vi "spectrum-voice.vi"() -> ()   [LabVIEW 2016]
doc: "This VI configures your sound card for both input and output. On a Macintosh, it could be the same device, while on Windows, it has to be different. Because of the delay of data buffering, it creates an effect of echoing."
uses:
  <vilib>/sound2/lvsound2.llb/Sound Data Format.ctl
  <vilib>/Analysis/3filter.llb/IIR Cascade Filter with I.C. (DBL).vi
  <vilib>/sound2/lvsound2.llb/Sound Input Read (DBL).vi
  <vilib>/express/express analysis/Spectral/Block/exnSpectralBlock spectral measurements power poly.vi
  <vilib>/express/express analysis/Spectral/Block/exnSpectralBlock spectral measurements power DDT.vi
  <vilib>/sound2/lvsound2.llb/Sound Output Write (DBL Single).vi
  <vilib>/express/express analysis/Spectral/XNode/ExpressSpectralMeasurementsBlockNode.xnode
  <vilib>/Analysis/NI_AALBase.lvlib
panel:
  in  "device ID":u32
  in  "Microphone\nAmplification":dbl(knob)=24.0 scale=0.0..100.0
  out "Time-Domain (Oscilloscope) Display":waveform(dbl)(graph)
  out "Frequency Display":dynamicdata(graph)
  in  "Filter":bool
  in  "filter type":T1(ring)
  in  "stop":bool
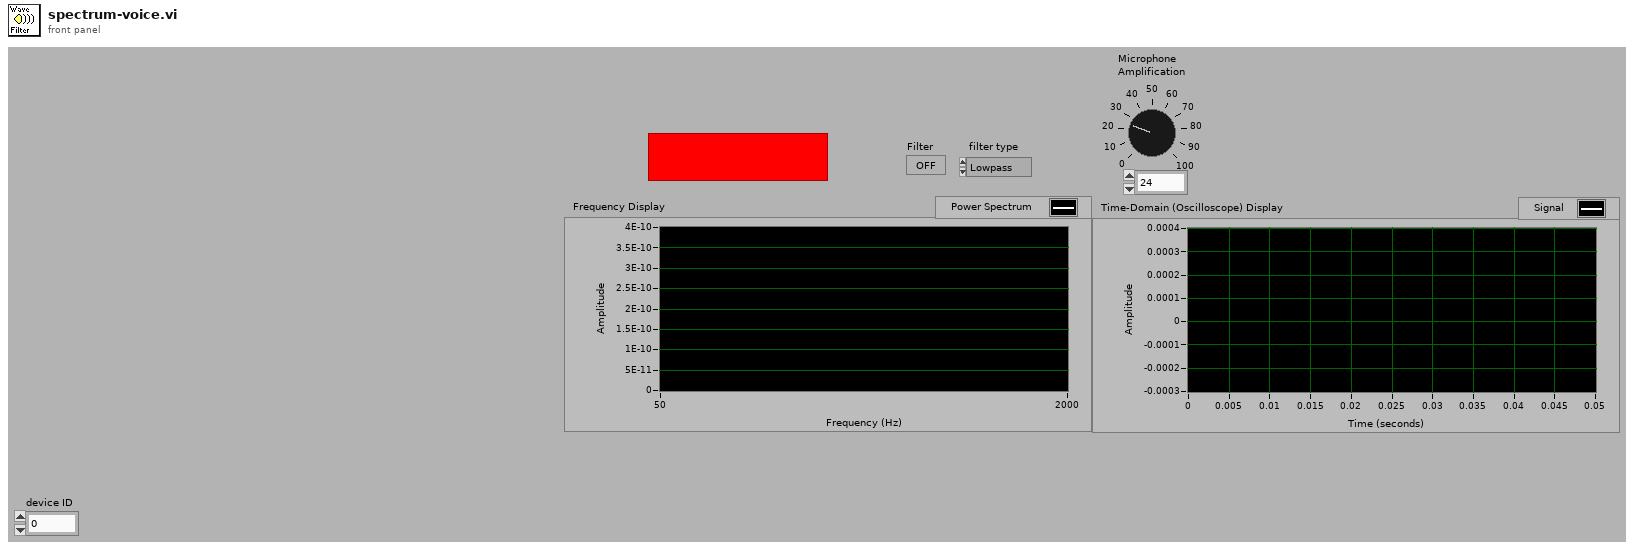
[diagram p1: front panel]
types:
  T1 = enum32{"Lowpass", "Highpass", "Bandpass", "Bandstop"}
  T2 = typedef "Sound Data Format.ctl" = cluster{"sample rate (S/s)":dbl, "number of channels":i32, "bits per sample":i32}
  T3 = typedef "Sound Output Task ID.ctl" = u32
  T4 = typedef "Sound Input Task ID.ctl" = u32
  T5 = cluster{"averaging mode":u16, "weighting mode":u16, "number of averages":u32}
  T6 = cluster{"dB On (F)":bool, "unwrap phase (F)":bool, "convert to degree (F)":bool}
  T7 = cluster{"filter structure":enum32{"IIR 2nd Order", "IIR 4th Order"}, "Reverse Coefficients":dbl[], "Forward Coefficients":dbl[]}
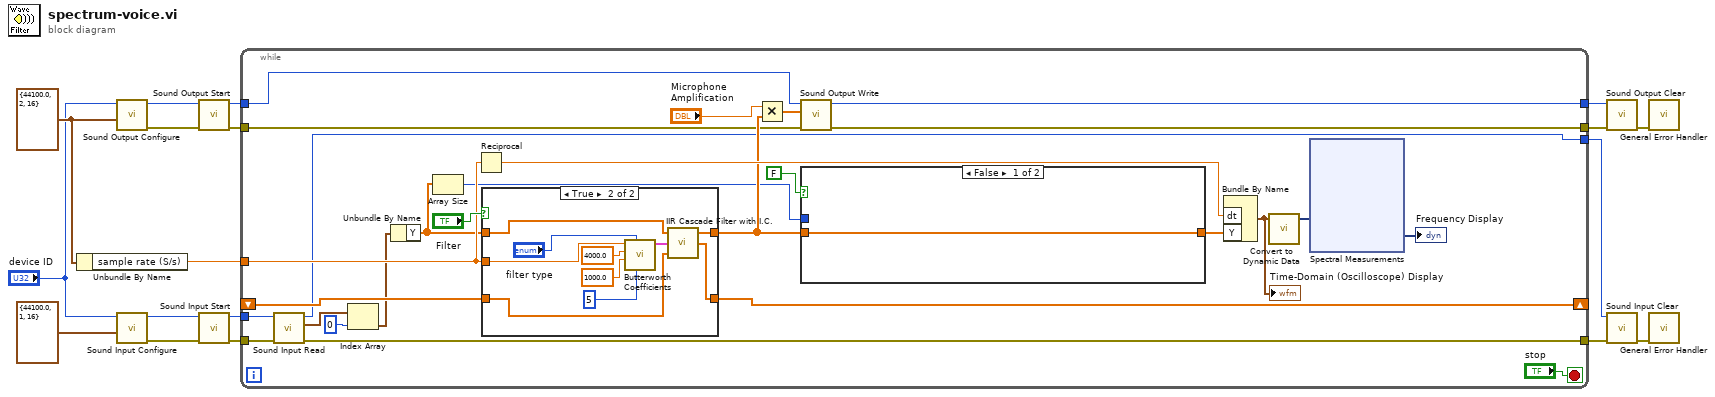
[diagram p0: block diagram]
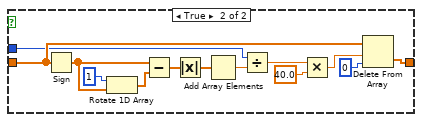
[diagram p2: hidden frame]
diagram:
  w14 = T2 {"sample rate (S/s)"=44100.0, "number of channels"=2, "bits per sample"=16} ("sound format")
  n1 = Unbundle By Name(w14) -> ("sample rate (S/s)"=w9:dbl)
  n2 = call <vilib>:"Sound Output Configure.vi"("sound format"=w14, "device ID"="device ID") -> ("error out"=w15:errorcluster, "task ID"=w16:T3)  [unwired: 8 in]
  n3 = call <vilib>:"Sound Input Configure.vi"("sound format"=T2 {"sample rate (S/s)"=44100.0, "number of channels"=1, "bits per sample"=16}, "device ID"="device ID") -> ("error out"=w18:errorcluster, "task ID"=w17:T4)  [unwired: 8 in]
  n4 = call <vilib>:"Sound Output Start.vi"("error in (no error)"=w15, "task ID"=w16) -> ("error out"=w8:errorcluster, "task ID out"=w7:T3)  [unwired: 8 in]
  n5 = call <vilib>:"Sound Input Start.vi"("error in (no error)"=w18, "task ID"=w17) -> ("error out"=w10:errorcluster, "task ID out"=w11:T4)  [unwired: 8 in]
  n6 = while {
    tunnel: w7 -> [w30]
    tunnel: w8 -> [w29]
    tunnel: [w26] -> w5
    tunnel: [w27] -> w6
    tunnel: w10 -> [w32]
    tunnel: [w24] -> w3
    tunnel: [w25] -> w2
    shift-right: [w44] -> _
    shift-left: _ -> [w43]
    tunnel: w9 -> [w39]
    tunnel: w11 -> [w31]
    stop <- "stop" stop-if-true
    n7 = call-poly <vilib>:"Sound Input Read.vi"("error in (no error)"=w32, "task ID"=w31) -> ("error out"=w25:errorcluster, "data"=w23:waveform(dbl)[], "task ID out"=w24:T4)  [unwired: 7 in]
    n8 = Index Array(array=w23, index=0) -> (element=w21:waveform(dbl))
    n9 = Unbundle By Name(w21) -> ("Y"=w22:dbl[])
    n10 = Array Size(array=w22) -> (size(s)=w33:i32)
    n11 = Reciprocal(x=w39) -> (1/x=w40:dbl)
    n12 = case shown="True" "Filter" {
      tunnel: [w70 w77] -> w35
      tunnel: w22 -> [w70 w76]
      tunnel: [w69 w75] -> w44
      tunnel: w43 -> [w69 w74]
      tunnel: w39 -> [_ w72]
      frame False {
      }
      frame True {
        n13 = call <vilib>:"Butterworth Coefficients.vi"("order"=5, "filter type"="filter type", "low cutoff freq: fl"=1000.0, "high cutoff freq: fh"=4000.0, "sampling freq: fs"=w72) -> ("IIR Filter Cluster"=w80:T7)  [unwired: 5 in, 1 out]
        n14 = call-poly <vilib>:"IIR Cascade Filter with I.C..vi"("Initial Filter State"=w74, "IIR Filter Cluster"=w80, "X"=w76) -> ("Final Filter State"=w75:dbl[], "Filtered X"=w77:dbl[])  [unwired: 1 out]
      }
    }
    n15 = Multiply(x="Microphone\nAmplification", y=w35) -> (x*y=w28:dbl[])
    n16 = call-poly <vilib>:"Sound Output Write.vi"("error in (no error)"=w29, "data"=w28, "task ID"=w30) -> ("error out"=w26:errorcluster, "task ID out"=w27:T3)  [unwired: 7 in]
    n17 = case shown="False" FALSE {
      tunnel: w35 -> [w46 w53]
      tunnel: [w46 w52] -> w34
      tunnel: w33 -> [_ w51]
      frame False {
      }
      frame True {
        n18 = Sign(1:w53) -> (0:w58:dbl[])
        n19 = Rotate 1D Array(1:w58, 2:1 ("n")) -> (0:w57:dbl[])
        n20 = Subtract(x=w58, y=w57) -> (x-y=w56:dbl[])
        n21 = Absolute Value(x=w56) -> (abs(x)=w55:dbl[])
        n22 = Add Array Elements(numeric array=w55) -> (sum=w50:dbl)
        n23 = Divide(x=w51, y=w50) -> (x/y=w48:dbl)
        n24 = Multiply(x=w48, y=40.0) -> (x*y=w47:dbl)
        n25 = Delete From Array(array=w53, length=w47, index=0) -> (deleted portion=w52:dbl[])  [unwired: 1 out]
      }
    }
    n26 = Bundle By Name("dt"=w40, "Y"=w34) -> (w38:waveform(dbl))  [unwired: 1 in]
    "Time-Domain (Oscilloscope) Display" <- w38
    n27 = call "Convert to Dynamic Data"("Waveform"=w38) -> ("Dynamic Data Type"=w37:dynamicdata)  [unwired: 3 in]
    n28 = xnode "Spectral Measurements"("Signals"=w37) -> ("Power Spectrum"=→"Frequency Display":dynamicdata)  [unwired: 1 in, 1 out]
  }
  n29 = call <vilib>:"Sound Output Clear.vi"("error in (no error)"=w5, "task ID"=w6) -> ("error out"=w4:errorcluster)  [unwired: 9 in]
  n30 = call <vilib>:"Sound Input Clear.vi"("error in (no error)"=w2, "task ID"=w3) -> ("error out"=w1:errorcluster)  [unwired: 9 in]
  n31 = call <vilib>:"General Error Handler.vi"("error in (no error)"=w4) -> ()  [unwired: 10 in, 5 out]
  n32 = call <vilib>:"General Error Handler.vi"("error in (no error)"=w1) -> ()  [unwired: 10 in, 5 out]
